vi "Create.vi"(8 "error in (no error)":errorcluster, 9 "Top VI":refnum<vi>, 10 "Listbox":refnum<vi>, 11 "Index":i32) -> (0 "error out":errorcluster, 3 "reference out":refnum<class "Multi Column Listbox.lvclass">)   [LabVIEW 2013, in "Table Manager.lvlib" / "Multi Column Listbox.lvclass"]
uses:
  Multi Column Listbox.lvclass
  Multi Column Listbox.lvclass/Multi Column Listbox.ctl
  Table Manager/Table Manager.lvclass/Table Manager.ctl
  Write Listbox.vi
  Table Manager/Write Index.vi
  Table Manager/Write Top VI.vi
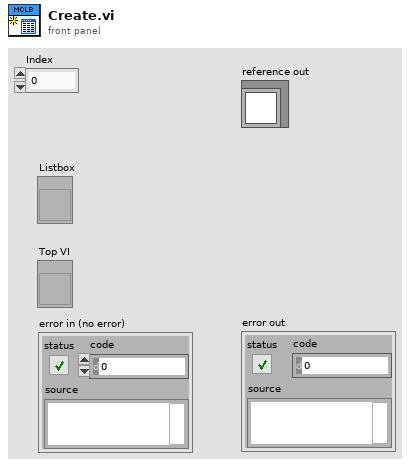
[diagram p1: front panel]
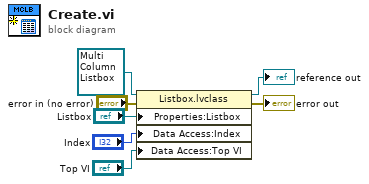
[diagram p0: block diagram]
diagram:
  n1 = property class="Listbox.lvclass"(reference=refnum<class "Multi Column Listbox.lvclass"> refnum ("Table Manager.lvlib:Multi Column Listbox.lvclass"), error in="error in (no error)", "Properties:Listbox"="Listbox", "Data Access:Index"="Index", "Data Access:Top VI"="Top VI") -> (reference out=→"reference out":refnum<class "Multi Column Listbox.lvclass">, error out=→"error out":errorcluster)
